vi "Analog Out Control.vi"(0 "VISA resource name":refnum<visa-resource-name>, 1 "Pin":u8 max=7 step=1, 2 "duty cycle":i16, 3 "error in (no error)":errorcluster) -> (7 "VISA resource name out":refnum<visa-resource-name>, 10 "error out":errorcluster)   [LabVIEW 2022 SP3, in "usbtmc_scpi_labtool.lvlib"]
doc: "Enables or Disables the output of power supply.\n\n* Output Enable (T:Enable) : \n If true it Switches ON the power supply Output else doesn't respond."
uses:
  usbtmc_scpi_labtool.lvlib
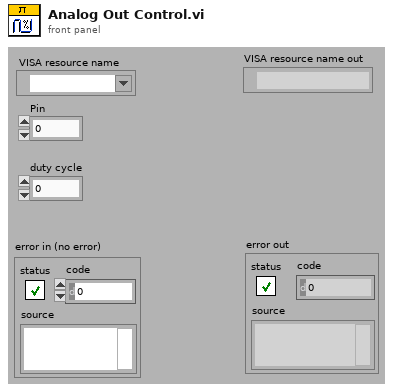
[diagram p1: front panel]
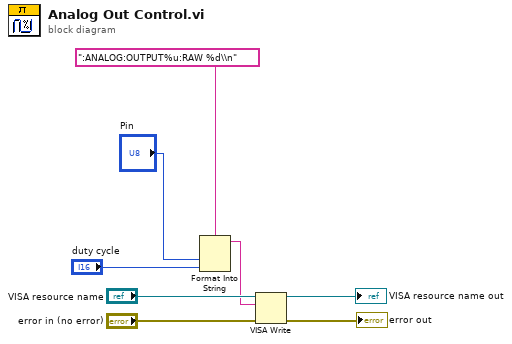
[diagram p0: block diagram]
diagram:
  n1 = Format Into String(format string=":ANALOG:OUTPUT%u:RAW %d\\n", "Pin", "duty cycle") -> (resulting string=w5:string)  [unwired: 2 in, 1 out]
  n2 = VISA Write(VISA resource name="VISA resource name", write buffer=w5, error in (no error)="error in (no error)") -> (VISA resource name out=→"VISA resource name out":refnum<visa-resource-name>, error out=→"error out":errorcluster)  [unwired: 1 out]
